vi "Measure current now.vi"() -> (3 "Current":dbl)   [LabVIEW 2011]
uses:
  <instrlib>/keithley_24xx/Keithley 24XX/Public/Data/Read (Single Point).vi
  <instrlib>/keithley_24xx/Keithley 24XX/Keithley 24XX.lvlib
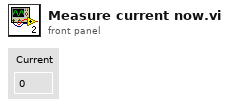
[diagram p1: front panel]
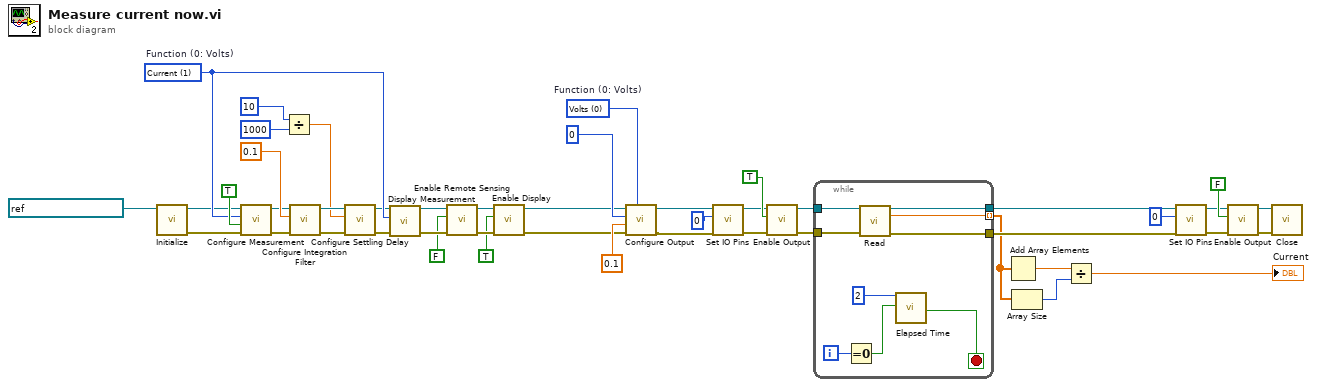
[diagram p0: block diagram]
diagram:
  w14 = u16 0 items=["Volts", "Current", "Resistance"]  # Function (0: Volts)
  w41 = u16 1 items=["Volts", "Current", "Resistance"]  # Function (0: Volts)
  n1 = call <instrlib>:"Initialize.vi"("VISA resource name"=refnum<visa-resource-name> "GPIB0::24::INSTR") -> ("error out"=w31:errorcluster, "VISA resource name out"=w32:refnum<visa-resource-name>)  [unwired: 4 in, 5 out]
  n2 = call <instrlib>:"Configure Measurement.vi"("error in (no error)"=w31, "Enable Auto Range (T:Enable)"=TRUE, "Function (0: Volts)"=w41, "VISA resource name"=w32) -> ("error out"=w34:errorcluster, "VISA resource name out"=w33:refnum<visa-resource-name>)  [unwired: 6 in]
  n3 = Divide(x=10, y=1000) -> (x/y=w40:dbl)
  n4 = call <instrlib>:"Configure Integration Filter.vi"("error in (no error)"=w34, "Measurement Speed (1 PLC)"=0.1, "VISA resource name"=w33) -> ("error out"=w43:errorcluster, "VISA resource name out"=w42:refnum<visa-resource-name>)  [unwired: 7 in]
  n5 = call <instrlib>:"Configure Settling Delay.vi"("error in (no error)"=w43, "Manual Settling Delay (0 sec)"=w40, "VISA resource name"=w42) -> ("error out"=w38:errorcluster, "VISA resource name out"=w37:refnum<visa-resource-name>)  [unwired: 7 in]
  n6 = call <instrlib>:"Display Measurement.vi"("error in (no error)"=w38, "Displayed Measurement (0: Voltage)"=w41, "VISA resource name"=w37) -> ("error out"=w36:errorcluster, "VISA resource name out"=w35:refnum<visa-resource-name>)  [unwired: 7 in]
  n7 = call <instrlib>:"Enable Remote Sensing.vi"("error in (no error)"=w36, "Enable Remote Sensing (T: Enable)"=FALSE, "VISA resource name"=w35) -> ("error out"=w29:errorcluster, "VISA resource name out"=w30:refnum<visa-resource-name>)  [unwired: 7 in]
  n8 = call <instrlib>:"Enable Display.vi"("error in (no error)"=w29, "Enable Display (T: Enable)"=TRUE ("Enable Output (T: Enable)"), "VISA resource name"=w30) -> ("error out"=w1:errorcluster, "VISA resource name out"=w2:refnum<visa-resource-name>)  [unwired: 7 in]
  n9 = call <instrlib>:"Configure Output.vi"("Source Mode  (0: Voltage)"=w14, "error in (no error)"=w1, "Compliance  Level (0.1)"=0.1 ("Compliance  Level"), "Output Level (0)"=0, "VISA resource name"=w2) -> ("error out"=w5:errorcluster, "VISA resource name out"=w6:refnum<visa-resource-name>)  [unwired: 5 in]
  n10 = call <instrlib>:"Set IO Pins.vi"("error in (no error)"=w5, "Output Pattern (0)"=0 ("Numeric"), "VISA resource name"=w6) -> ("error out"=w3:errorcluster, "VISA resource name out"=w4:refnum<visa-resource-name>)  [unwired: 7 in]
  n11 = call <instrlib>:"Enable Output.vi"("error in (no error)"=w3, "Enable Output (T: Enable)"=TRUE ("Output (Off)"), "VISA resource name"=w4) -> ("error out"=w24:errorcluster, "VISA resource name out"=w25:refnum<visa-resource-name>)  [unwired: 7 in]
  n12 = while {
    tunnel: w25 -> [w55]
    tunnel: w24 -> [w54]
    tunnel: [w53] -> w19
    tunnel: [w51] -> w11 mode=indexing
    tunnel: [w47] -> w16
    i -> [w50]
    stop <- w52 stop-if-true
    n13 = Equal To 0?(x=w50) -> (x = 0?=w49:bool)
    n14 = call-poly <instrlib>:"Read.vi"("VISA resource name"=w55, "error in (no error)"=w54) -> ("VISA resource name out"=w53:refnum<visa-resource-name>, "Current"=w51:sgl, "error out"=w47:errorcluster)  [unwired: 7 in, 4 out]
    n15 = call "Elapsed Time"("Time Target (s)"=2, "Reset"=w49) -> ("Time has Elapsed"=w52:bool)  [unwired: 10 in, 7 out]
  }
  n16 = Add Array Elements(numeric array=w11) -> (sum=w12:sgl)
  n17 = Array Size(array=w11) -> (size(s)=w10:i32)
  n18 = Divide(x=w12, y=w10) -> (x/y=→"Current":sgl)
  n19 = call <instrlib>:"Set IO Pins.vi"("error in (no error)"=w16, "Output Pattern (0)"=0, "VISA resource name"=w19) -> ("error out"=w15:errorcluster, "VISA resource name out"=w20:refnum<visa-resource-name>)  [unwired: 7 in]
  n20 = call <instrlib>:"Enable Output.vi"("error in (no error)"=w15, "Enable Output (T: Enable)"=FALSE ("Output (Off)"), "VISA resource name"=w20) -> ("error out"=w22:errorcluster, "VISA resource name out"=w23:refnum<visa-resource-name>)  [unwired: 7 in]
  n21 = call <instrlib>:"Close.vi"("error in (no error)"=w22, "VISA resource name"=w23) -> ()  [unwired: 9 in, 1 out]
